vi "Read Reg DAQ Racks.vi"(0 "Reg DAQ Rack Path":path, 1 "Cal Base Path":path) -> (15 "Registered Systems":T1[](array[typedef]), 19 "error out":errorcluster)   [LabVIEW 2019]
uses:
  Type Defs and Controls/Registered System.ctl
  Type Defs and Controls/System Type.ctl
  <vilib>/Utility/config.llb/Read Key (String).vi
  <vilib>/Utility/config.llb/NI_LVConfig.lvlib
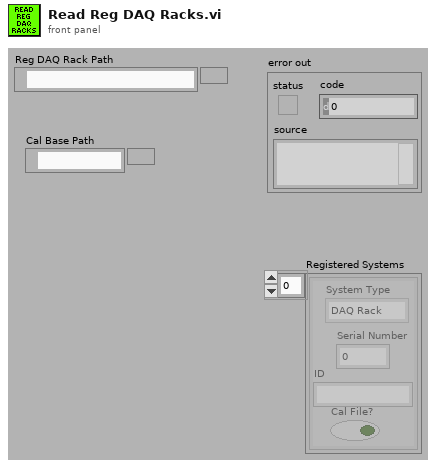
[diagram p1: front panel]
types:
  T1 = typedef "Registered System.ctl" = cluster{"System Type":T2, "Serial Number":u32, "ID":string, "Cal File?":bool}
  T2 = typedef "System Type.ctl" = enum16{"DAQ Rack", "DAQ Cart", "nx-5000", "unknown", "open"}
  T3 = typedef "NI_LVConfig.lvlib/Config Data RefNum.ctl" = refnum<k1>
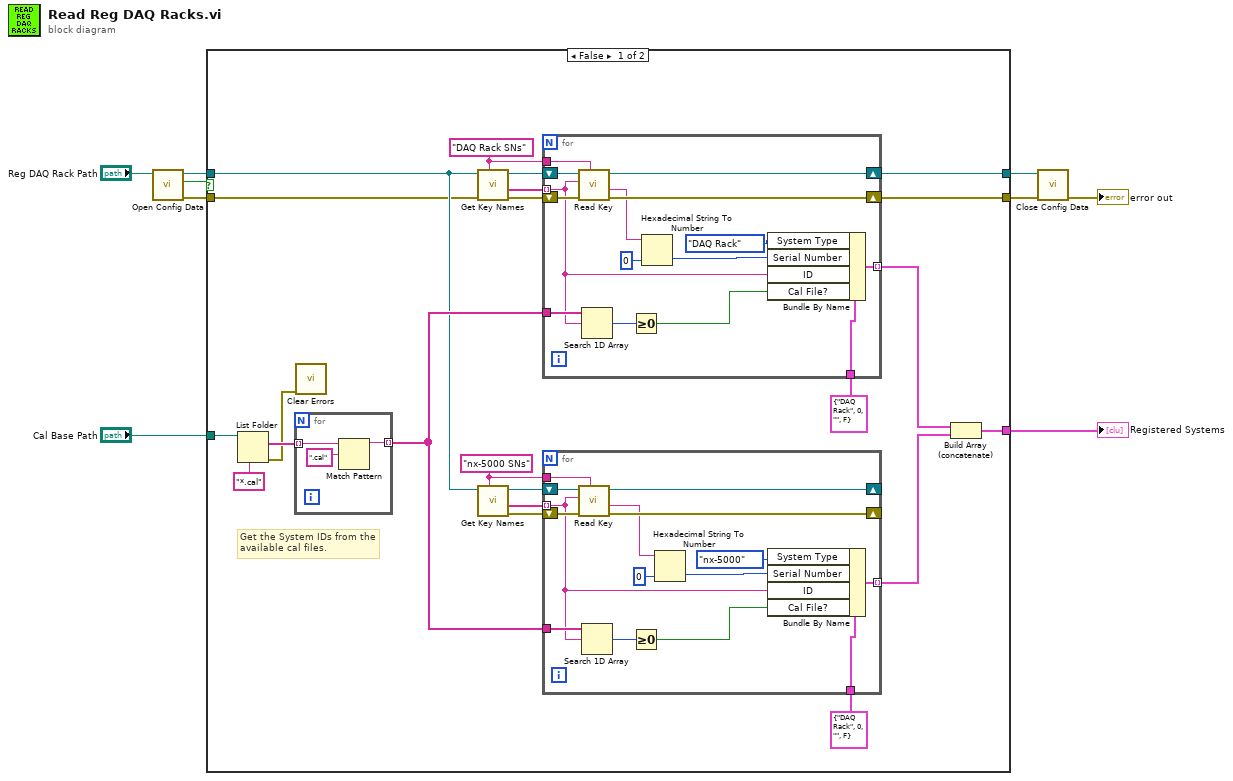
[diagram p0: block diagram]
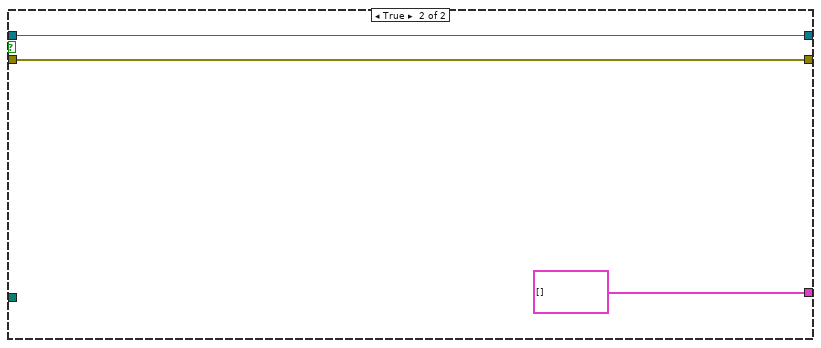
[diagram p2: hidden frame]
diagram:
  n1 = call <vilib>:"Open Config Data.vi"("configuration file path"="Reg DAQ Rack Path") -> ("error out"=w4:errorcluster, "file created?"=w8:bool, "refnum"=w5:T3)  [unwired: 8 in]
  n2 = case shown="False" w8 {
    tunnel: w4 -> [w14 w65]
    tunnel: w5 -> [w15 w66]
    tunnel: [w12 w65] -> w6
    tunnel: [w13 w66] -> w7
    tunnel: [w16 T1[] []] -> w2
    tunnel: "Cal Base Path" -> [w11 _]
    frame False {
      w20 = "nx-5000 SNs" ("section")
      w31 = "DAQ Rack SNs" ("section")
      # "Get the System IDs from the \navailable cal files."
      n3 = List Folder(path=w11, pattern="*.cal" ("string")) -> (filenames=w27:string[], error out=w10:errorcluster)  [unwired: 2 in, 2 out]
      n4 = for {
        tunnel: w27 -> [w49] mode=indexing
        tunnel: [w48] -> w19 mode=indexing
        n5 = Match Pattern(string=w49, regular expression=".cal" ("string")) -> (before substring=w48:string)  [unwired: 1 in, 3 out]
      }
      n6 = call <vilib>:"Clear Errors.vi"("error in (no error)"=w10) -> ()  [unwired: 5 in, 2 out]
      n7 = call <vilib>:"Get Key Names.vi"("section"=w31, "error in (no error)"=w14, "refnum"=w15) -> ("error out"=w29:errorcluster, "key names"=w30:string[], "refnum out"=w28:T3)  [unwired: 5 in, 1 out]
      n8 = call <vilib>:"Get Key Names.vi"("section"=w20, "refnum"=w15) -> ("error out"=w22:errorcluster, "key names"=w21:string[], "refnum out"=w23:T3)  [unwired: 6 in, 1 out]
      n9 = for {
        tunnel: w31 -> [w64]
        tunnel: w30 -> [w54] mode=indexing
        shift-right: [w62] -> w12
        shift-left: w29 -> [w63]
        shift-right: [w60] -> w13
        shift-left: w28 -> [w61]
        tunnel: T1 {"System Type"=enum."DAQ Rack", "Serial Number"=0, "ID"="", "Cal File?"=FALSE} ("Cluster") -> [w57]
        tunnel: w19 -> [w55]
        tunnel: [w51] -> w18 mode=indexing
        n10 = call-poly <vilib>:"Read Key.vi"("section"=w64, "error in (no error)"=w63, "key"=w54, "refnum"=w61) -> ("error out"=w62:errorcluster, "value"=w59:string, "refnum out"=w60:T3)  [unwired: 4 in, 1 out]
        n11 = Search 1D Array(1D array=w55, element=w54) -> (index of element=w53:i32)  [unwired: 1 in]
        n12 = Greater Or Equal To 0?(x=w53) -> (x >= 0?=w52:bool)
        n13 = Hexadecimal String To Number(string=w59, default (0uL)=u32 0 ("default (0 U32)")) -> (number=w56:u32)  [unwired: 1 in, 1 out]
        n14 = Bundle By Name(cluster=w57, "System Type"=System_Type."DAQ Rack", "Serial Number"=w56, "ID"=w54, "Cal File?"=w52) -> (w51:T1)
      }
      n15 = for {
        tunnel: w20 -> [w46]
        tunnel: w21 -> [w36] mode=indexing
        shift-right: [w44] -> _
        shift-left: w22 -> [w45]
        shift-right: [w42] -> _
        shift-left: w23 -> [w43]
        tunnel: T1 {"System Type"=enum."DAQ Rack", "Serial Number"=0, "ID"="", "Cal File?"=FALSE} ("Cluster") -> [w39]
        tunnel: w19 -> [w37]
        tunnel: [w33] -> w17 mode=indexing
        n16 = call-poly <vilib>:"Read Key.vi"("section"=w46, "error in (no error)"=w45, "key"=w36, "refnum"=w43) -> ("error out"=w44:errorcluster, "value"=w41:string, "refnum out"=w42:T3)  [unwired: 4 in, 1 out]
        n17 = Search 1D Array(1D array=w37, element=w36) -> (index of element=w35:i32)  [unwired: 1 in]
        n18 = Greater Or Equal To 0?(x=w35) -> (x >= 0?=w34:bool)
        n19 = Hexadecimal String To Number(string=w41, default (0uL)=u32 0 ("default (0 U32)")) -> (number=w38:u32)  [unwired: 1 in, 1 out]
        n20 = Bundle By Name(cluster=w39, "System Type"=System_Type."nx-5000", "Serial Number"=w38, "ID"=w36, "Cal File?"=w34) -> (w33:T1)
      }
      n21 = Build Array (concatenate)(w18, w17) -> (w16:T1[])
    }
    frame True {
    }
  }
  "Registered Systems" <- w2
  n22 = call <vilib>:"Close Config Data.vi"("error in (no error)"=w6, "refnum"=w7) -> ("error out"=→"error out":errorcluster)  [unwired: 8 in, 1 out]
